vi "Numeric Indicator (Silver).vi"() -> ()   [LabVIEW 2012]
panel:
  out "Numeric Indicator":dbl
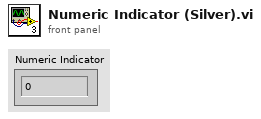
[diagram p1: front panel]
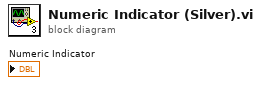
[diagram p0: block diagram]
diagram:
